vi "PCAN_INIT.vi"(7 "path in":path, 8 "error in (no error)":errorcluster, 10 "Msg Type":i32(ring) items=["standart", "extended"], 11 "BTR0BTR1":u16(ring)=20 items=["1M"=20, "500K"=28, "250K"=284, "125K"=796, "100K"=17199, "50K"=18223, "20K"=21295, "10K"=26415, "5K"=32639]) -> (0 "error out":errorcluster, 2 "path out":path, 3 "error":T1 items=["CAN_ERR_OK"=0, "CAN_ERR_XMTFULL"=1, "CAN_ERR_OVERRUN"=2, "CAN_ERR_BUSLIGHT"=4, "CAN_ERR_BUSHEAVY"=8, "CAN_ERR_BUSOFF"=16, "CAN_ERR_QRCVEMPTY"=32, "CAN_ERR_QOVERRUN"=64, "CAN_ERR_QXMTFULL"=128, "CAN_ERR_REGTEST"=256, "CAN_ERR_NOVXD"=512, "CAN_ERR_HWINUSE"=1024, "CAN_ERR_NETINUSE"=2048, "CAN_ERR_ILLHW"=5120, "CAN_ERR_ILLNET"=6144, "CAN_ERR_ILLCLINET"=7168, "CAN_ERR_RESOURCE"=8192, "CAN_ERR_ILLPARAMTYPE"=16384, "CAN_ERR_ILLPARAMVAL"=32768, "CAN_ERR_UNKNOWN"=65536])   [LabVIEW 2019]
doc: "///////////////////////////////////////////////////////////////////////////////\n// CAN_Init()\n// Aktiviert eine Hardware, macht Registertest des 82C200/SJA1000,\n// teilt einen Sendepuffer und ein HardwareHandle zu.\n// Programmiert Konfiguration der Sende/Empfangstreiber.\n// Controller bleibt im Resetzustand.\n// Uebergibt die Baudratenregister\n// Wenn CANMsgType=0 ---> 11Bit ID Betrieb\n// Wenn CANMsgType=1 ---> 11/29Bit ID Betrieb\n// moegliche Fehler: NOVXD ILLHW REGTEST RESOURCE\n// \n\nDWORD __stdcall CAN_Init(WORD wBTR0BTR1, int CANMsgType); // Baudrate"
uses:
  controls/PCAN_ERROR.ctl
  PCAN_USB.dll
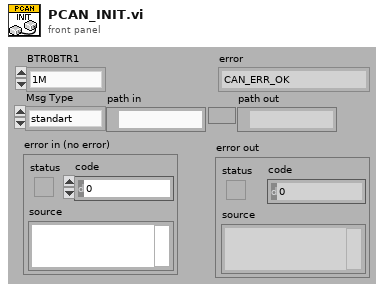
[diagram p1: front panel]
types:
  T1 = typedef "PCAN_ERROR.ctl" = i32
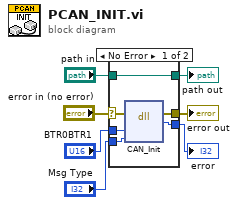
[diagram p0: block diagram]
diagram:
  n1 = case shown="No Error" "error in (no error)" {
    selector: "error in (no error)" -> [w10 w15]
    tunnel: "BTR0BTR1" -> [w13 _]
    tunnel: "Msg Type" -> [w12 _]
    tunnel: [w11 _] -> w5
    tunnel: [w9 w15] -> w3
    tunnel: "path in" -> [w8 w14]
    tunnel: [w8 w14] -> w1
    frame No Error {
      n2 = dll-call lib="D:/Project/ASBCT/SubVI/PCAN_USB.dll" fn="CAN_Init"(error in=w10, "wBTR0BTR1"=w13, "CANMsgType"=w12) -> (error out=w9:errorcluster, "return type"=w11:i32)  [unwired: 4 in, 1 out]
    }
    frame Error {
    }
  }
  "error" <- w5
  "error out" <- w3
  "path out" <- w1
